vi "Servo 3 Init.vi"() -> (0 "error out":errorcluster, 3 "Servo":T1)   [LabVIEW 2020]
uses:
  <vilib>/High Genius/HG_WSI_Tookit/Dependencies/Library/PWM/PWM.lvclass
  C:/Program Files (x86)/National Instruments/LabVIEW 2020/vi.lib/High Genius/HG_WSI_Tookit/Dependencies/Library/HG_LIB/HG_LIB.lvclass
  <vilib>/High Genius/HG_WSI_Tookit/Dependencies/Library/HG_LIB/HG_LIB.lvclass
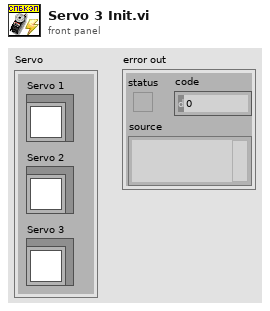
[diagram p1: front panel]
types:
  T1 = cluster{"Servo 1":refnum<class "PWM.lvclass">, "Servo 2":refnum<class "PWM.lvclass">, "Servo 3":refnum<class "PWM.lvclass">}
  T2 = enum16{"0", "1", "2", "3", "4", "5", "6", "7", "8", "9", "10", "11", "12", "13", "14", "15", "16", "17", "18", "19", "20", "21", "22", "23", "24", "25"}
  T3 = enum16{"DI", "DO", "AI", "Pulse", "PWM", "ISQ", "ENC", "CAN", "IIC", "IMU"}
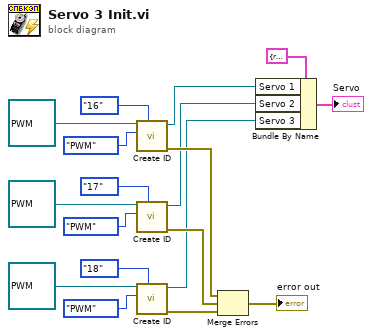
[diagram p0: block diagram]
diagram:
  n1 = call <vilib>:"Create ID.vi"("NO"=T2."16", "Function"=T3."PWM", "HG_LIB in"=refnum<class "PWM.lvclass"> refnum ("PWM.lvclass")) -> ("error out"=w7:errorcluster, "HG_LIB out"=w3:refnum<class "PWM.lvclass">)  [unwired: 7 in]
  n2 = call <vilib>:"Create ID.vi"("NO"=T2."17", "Function"=T3."PWM", "HG_LIB in"=refnum<class "PWM.lvclass"> refnum ("PWM.lvclass")) -> ("error out"=w8:errorcluster, "HG_LIB out"=w2:refnum<class "PWM.lvclass">)  [unwired: 7 in]
  n3 = call <vilib>:"Create ID.vi"("NO"=T2."18", "Function"=T3."PWM", "HG_LIB in"=refnum<class "PWM.lvclass"> refnum ("PWM.lvclass")) -> ("error out"=w9:errorcluster, "HG_LIB out"=w1:refnum<class "PWM.lvclass">)  [unwired: 7 in]
  n4 = Merge Errors(w7, w8, w9) -> (→"error out":errorcluster)
  n5 = Bundle By Name(cluster=T1 {"Servo 1"=refnum, "Servo 2"=refnum, "Servo 3"=refnum} ("HG_LIB out"), "Servo 1"=w3, "Servo 2"=w2, "Servo 3"=w1) -> (→"Servo":T1)
